vi "Read Inspect Module.vi"(8 "error in (no error)":errorcluster, 11 "Potting Procedure in":refnum<class "Potting Procedure.lvclass">) -> (0 "error out":errorcluster, 2 "Inspect Modules":T1, 3 "Potting Procedure out":refnum<class "Potting Procedure.lvclass">)   [LabVIEW 2011, in "Potting Procedure.lvclass"]
uses:
  Potting Procedure.lvclass
  Type Definitions/Inspect Modules.ctl
  Shared Components/Utils/Type Definitions/Multi-Fiducial Image.ctl
  Shared Components/Utils/Type Definitions/Physical Image.ctl
  Shared Components/Vec3d Class/Vec3d Class.lvclass
  <vilib>/vision/Image Controls.llb/IMAQ Image.ctl
  Shared Components/Utils/Type Definitions/Fiducial with Source.ctl
  Shared Components/Utils/Type Definitions/Fiducial Image.ctl
  Potting Procedure.lvclass/Potting Procedure.ctl
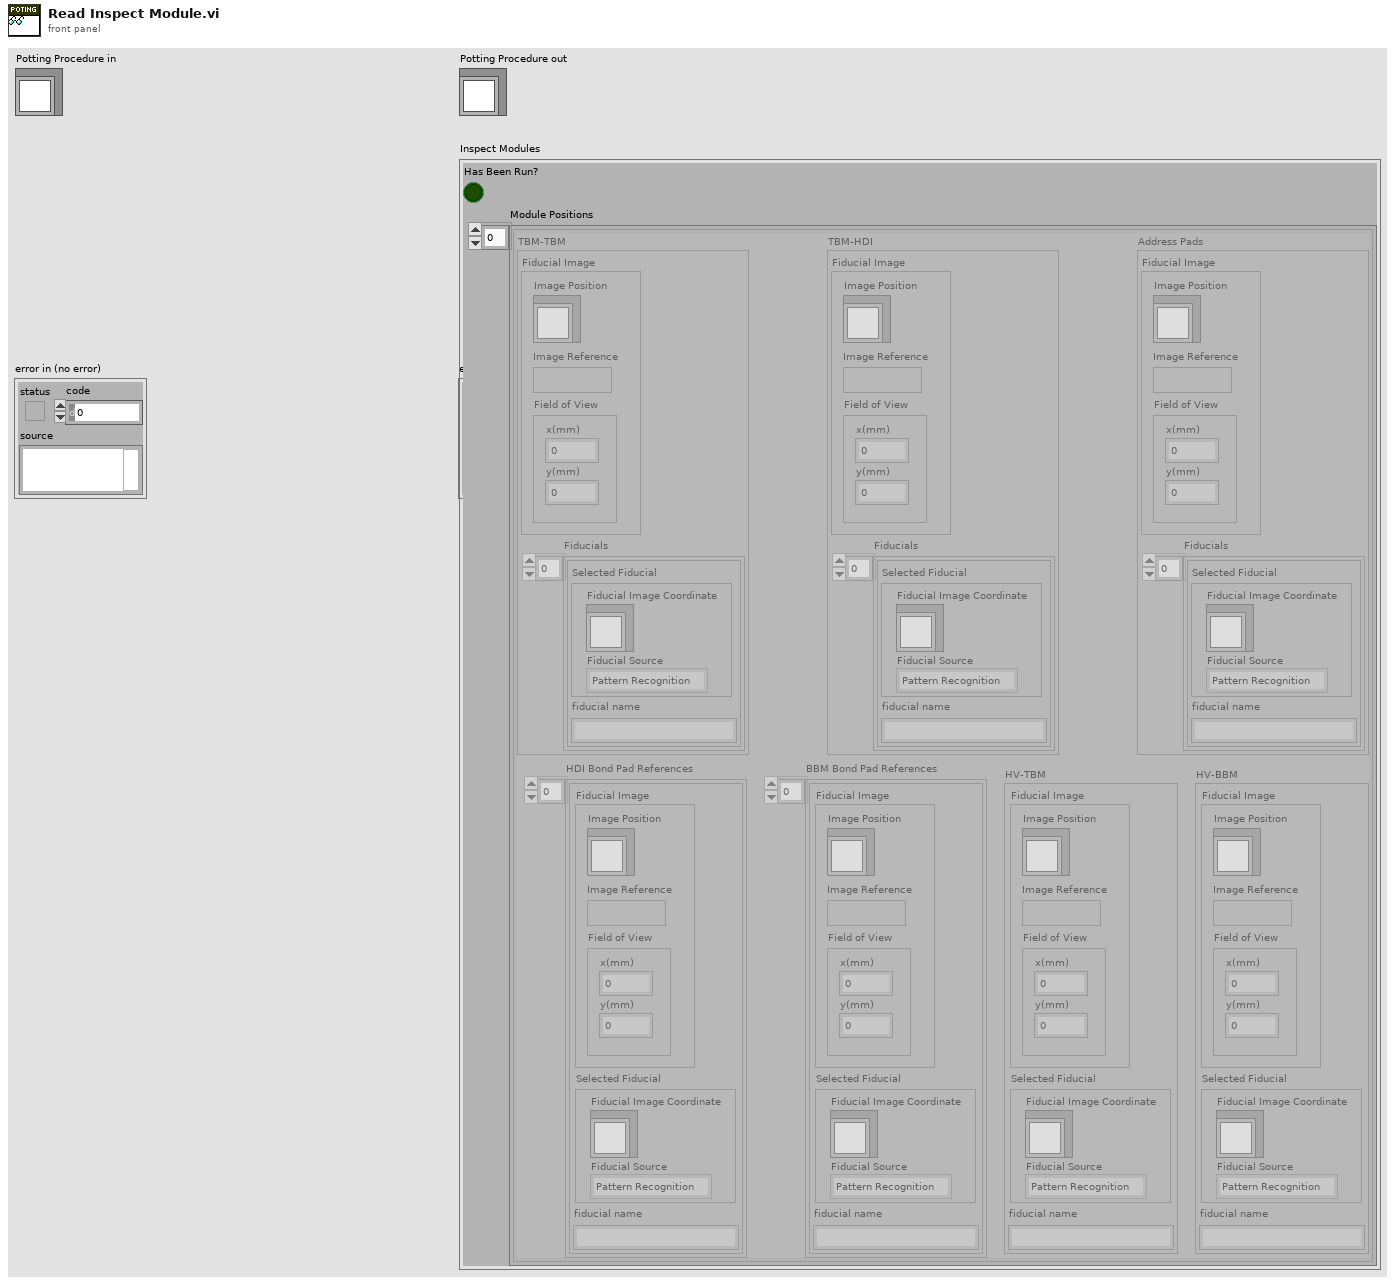
[diagram p1: front panel]
types:
  T1 = typedef "Inspect Modules.ctl" = cluster{"Has Been Run?":bool, "Module Positions":cluster{"TBM-TBM":T2, "TBM-HDI":T2, "Address Pads":T2, "HDI Bond Pad References":T6[], "BBM Bond Pad References":T6[], "HV-TBM":T6, "HV-BBM":T6}[]}
  T2 = typedef "Multi-Fiducial Image.ctl" = cluster{"Fiducial Image":T3, "Fiducials":cluster{"Selected Fiducial":T5, "fiducial name":string}[]}
  T3 = typedef "Physical Image.ctl" = cluster{"Image Position":refnum<class "Vec3d Class.lvclass">, "Image Reference":T4, "Field of View":cluster{"x(mm)":dbl, "y(mm)":dbl}}
  T4 = typedef "IMAQ Image.ctl" = refnum<image>
  T5 = typedef "Fiducial with Source.ctl" = cluster{"Fiducial Image Coordinate":refnum<class "Vec3d Class.lvclass">, "Fiducial Source":enum16{"Pattern Recognition", "User", "Error", "Default"}}
  T6 = typedef "Fiducial Image.ctl" = cluster{"Fiducial Image":T3, "Selected Fiducial":T5, "fiducial name":string}
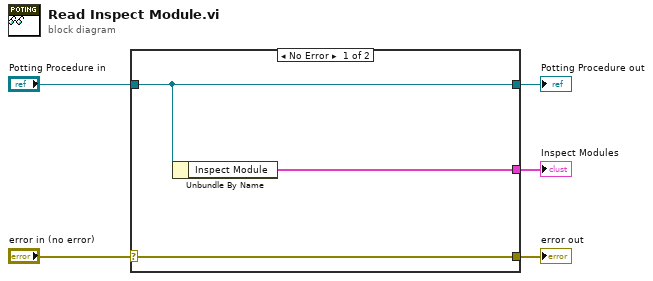
[diagram p0: block diagram]
diagram:
  n1 = case shown="No Error" "error in (no error)" {
    selector: "error in (no error)" -> [w8 w9]
    tunnel: [w8 w9] -> w4
    tunnel: [w7 w10] -> w2
    tunnel: "Potting Procedure in" -> [w7 w10]
    tunnel: [w6 _] -> w1
    frame No Error {
      n2 = Unbundle By Name(w7) -> ("Inspect Module"=w6:T1)
    }
    frame Error {
    }
  }
  "error out" <- w4
  "Potting Procedure out" <- w2
  "Inspect Modules" <- w1
